vi "Listening Server Cases.vi"(7 "Listening Queue":refnum<queue>, 8 "error in (no error)":errorcluster, 9 "Data":variant, 10 "Command":string, 11 "Generic Controller in":refnum<class "Generic Plugin.lvclass">) -> (0 "error out":errorcluster, 2 "Stop?":bool, 3 "Generic Controller out":refnum<class "Generic Plugin.lvclass">)   [LabVIEW 2020, in "RxnRover.lvlib" / "Generic Plugin.lvclass"]
doc: "Case structure with messages to listen for from the control panel. If more than the basic messages need to be handled, this should be overwritten by the child class."
uses:
  Generic Plugin.lvclass
  <userlib>/RxnRover/DynamicReentrant/src/Type Defs/Message.ctl
  Generic Plugin.lvclass/Generic Plugin.ctl
  events/Process Stopped Cluster.ctl
  Sub VIs/Message Queue/Enqueue Message (Single).vi
  RxnRover.lvlib
  Sub VIs/Message Queue/test Message Queue.lvlib
  <userlib>/RxnRover/DynamicReentrant/Dynamic Reentrant.lvlib
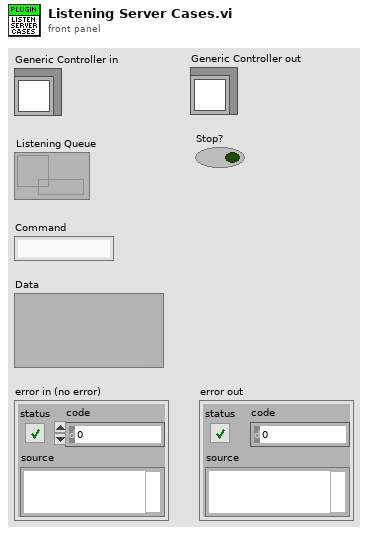
[diagram p1: front panel]
types:
  T1 = typedef "RxnRover.lvlib/Process Stopped Cluster.ctl" = cluster{"Name":string, "Type":enum16{"Hardware", "Optimizer", "Analyzer"}}
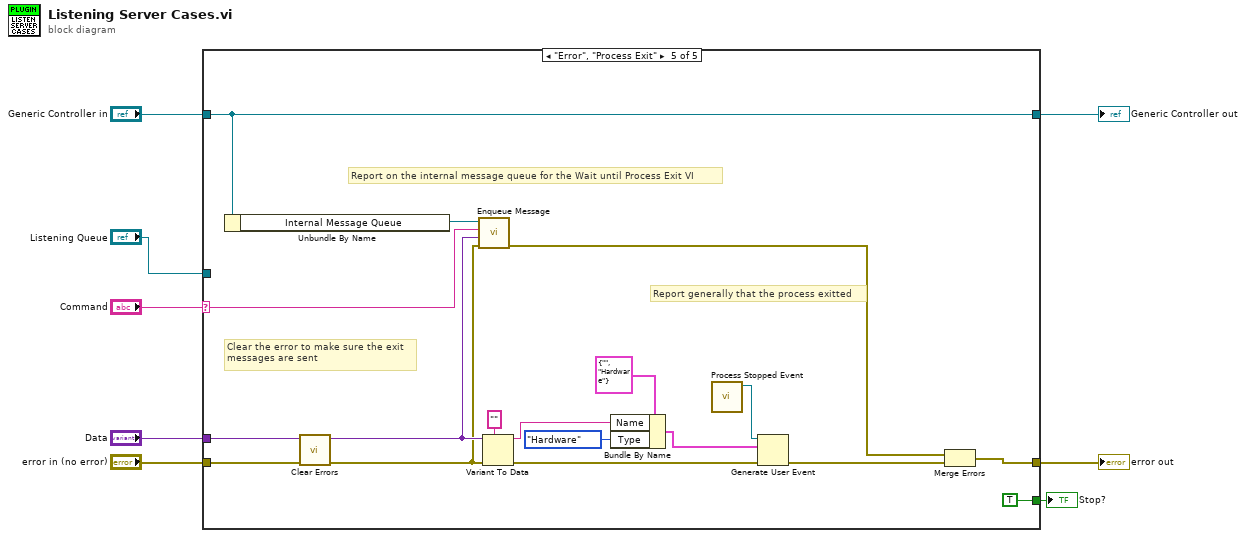
[diagram p0: block diagram]
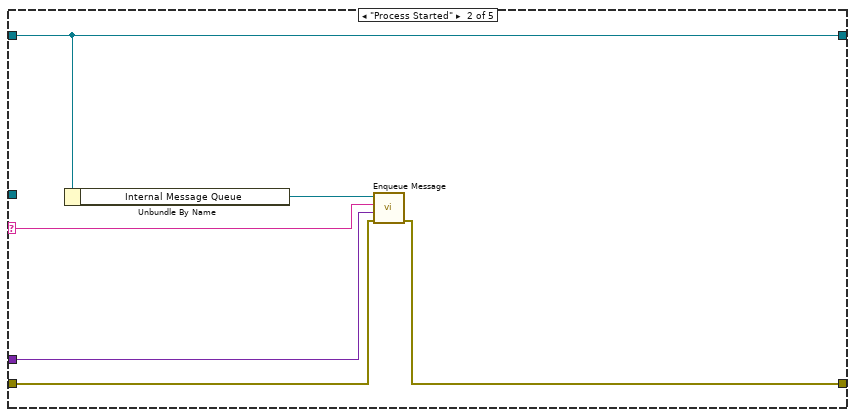
[diagram p3: hidden frame]
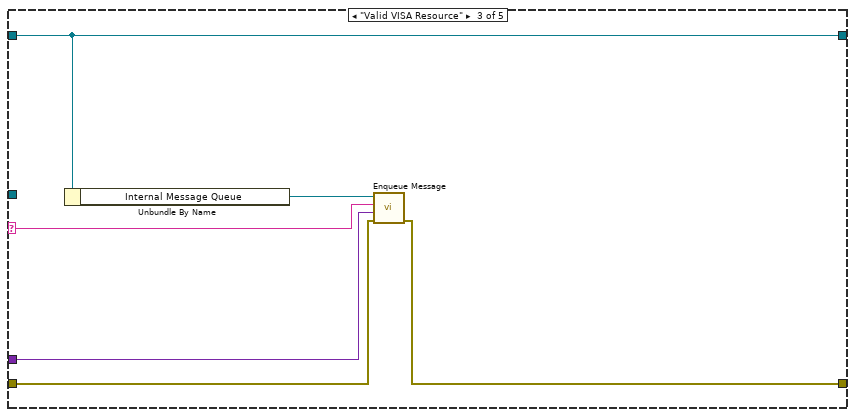
[diagram p4: hidden frame]
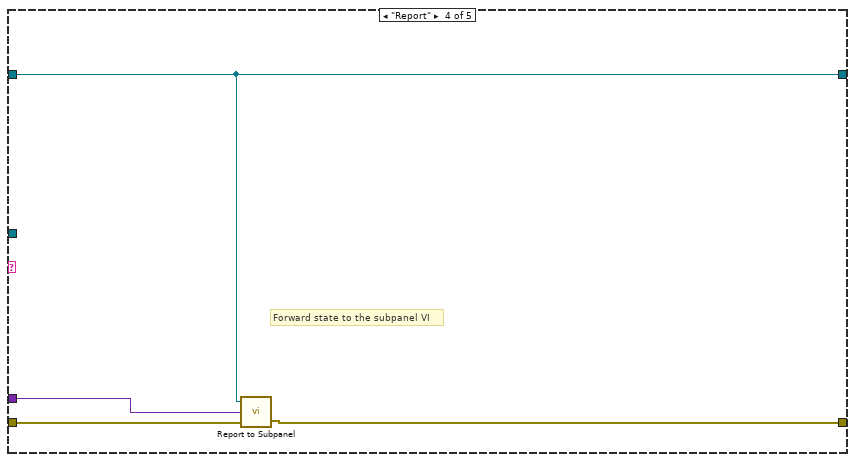
[diagram p5: hidden frame]
diagram:
  n1 = case shown="\"Error\", \"Process Exit\"" "Command" {
    selector: "Command" -> [_ w14 w20 _ w32]
    tunnel: "error in (no error)" -> [w9 w12 w18 w25 w30]
    tunnel: [w9 w11 w17 w24 w29] -> w2
    tunnel: "Generic Controller in" -> [w10 w16 w22 w23 w34]
    tunnel: [w10 w16 w22 w23 w34] -> w3
    tunnel: "Data" -> [_ w13 w19 w26 w31]
    tunnel: [_ _ _ _ TRUE] -> w8
    tunnel: "Listening Queue" -> [_ _ _ _ _]
    frame Default {
    }
    frame "Process Started" {
      n2 = Unbundle By Name(w16) -> ("Internal Message Queue"=w15:refnum<queue>)
      n3 = call-poly "Enqueue Message.vi"("error in (no error)"=w12, "Message Data"=w13, "Message"=w14, "Message Queue"=w15) -> ("error out"=w11:errorcluster)  [unwired: 6 in, 1 out]
    }
    frame "Valid VISA Resource" {
      n4 = Unbundle By Name(w22) -> ("Internal Message Queue"=w21:refnum<queue>)
      n5 = call-poly "Enqueue Message.vi"("error in (no error)"=w18, "Message Data"=w19, "Message"=w20, "Message Queue"=w21) -> ("error out"=w17:errorcluster)  [unwired: 6 in, 1 out]
    }
    frame "Report" {
      # "Forward state to the subpanel VI"
      n6 = call "Report to Subpanel.vi"("error in (no error)"=w25, "State"=w26, "controller in"=w23) -> ("error out"=w24:errorcluster)  [unwired: 1 out]
    }
    frame "Error", "Process Exit" {
      # "Clear the error to make sure the exit\nmessages are sent"
      # "Report generally that the process exitted"
      # "Report on the internal message queue for the Wait until Process Exit VI"
      n7 = Unbundle By Name(w34) -> ("Internal Message Queue"=w33:refnum<queue>)
      n8 = call <vilib>:"Clear Errors.vi"("error in (no error)"=w30) -> ("error out"=w27:errorcluster)  [unwired: 5 in, 1 out]
      n9 = call-poly "Enqueue Message.vi"("error in (no error)"=w27, "Message Data"=w31, "Message"=w32, "Message Queue"=w33) -> ("error out"=w28:errorcluster)  [unwired: 6 in, 1 out]
      n10 = Variant To Data(error in=w27, type="", Variant=w31) -> (data=w36:string, error out=w40:errorcluster)
      n11 = Bundle By Name(cluster=T1 {"Name"="", "Type"=enum."Hardware"} ("Process Cluster"), "Name"=w36, "Type"=enum16{"Hardware", "Optimizer"}."Hardware") -> (w37:T1)
      n12 = call "Process Stopped Event.vi"() -> ("Process Stopped"=w42:refnum<user-event>)  [unwired: 11 in]
      n13 = Generate User Event(user event=w42, event data cluster=w37, error in=w40) -> (error out=w41:errorcluster)  [unwired: 1 in, 1 out]
      n14 = Merge Errors(w28, w41) -> (w29:errorcluster)
    }
  }
  "Stop?" <- w8
  "Generic Controller out" <- w3
  "error out" <- w2
